vi "Record.vi"(8 "error in (no error)":errorcluster, 11 "Spectrum Recorder in":refnum<class "Spectrum Recorder.lvclass">) -> (0 "error out":errorcluster, 3 "Spectrum Recorder out":refnum<class "Spectrum Recorder.lvclass">)   [LabVIEW 2016, in "Spectrum Recorder.lvclass"]
uses:
  Spectrum Recorder.lvclass
  Spectrum Recorder.lvclass/Spectrum Recorder.ctl
  Red Pitaya/RP Core/RP Transceiver/RP Transceiver.lvclass
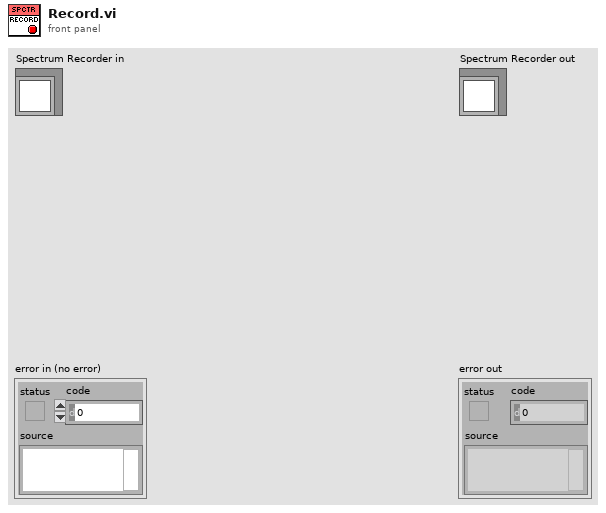
[diagram p1: front panel]
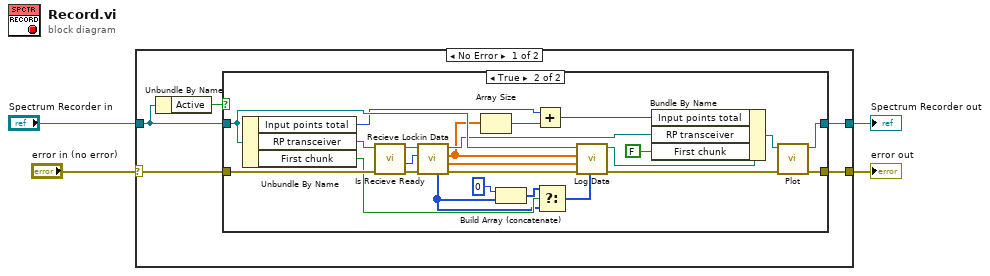
[diagram p0: block diagram]
diagram:
  n1 = case shown="No Error" "error in (no error)" {
    selector: "error in (no error)" -> [w6 w37]
    tunnel: [w5 w37] -> w3
    tunnel: [w7 w36] -> w1
    tunnel: "Spectrum Recorder in" -> [w8 w36]
    frame No Error {
      n2 = Unbundle By Name(w8) -> ("Active"=w9:bool)
      n3 = case shown="True" w9 {
        tunnel: w8 -> [w11 w28]
        tunnel: w6 -> [w10 w34]
        tunnel: [w11 w16] -> w7
        tunnel: [w10 w18] -> w5
        frame False {
        }
        frame True {
          n4 = Unbundle By Name(w28) -> ("Input points total"=w12:i64, "RP transceiver"=w35:refnum<class "RP Transceiver.lvclass">, "First chunk"=w27:bool)
          n5 = call-dynamic "Is Recieve Ready.vi"("error in (no error)"=w34, "RP Instrument in"=w35) -> ("error out"=w33:errorcluster, "Points in buffer"=w31:i32, "RP Instrument out"=w32:refnum<class "RP Transceiver.lvclass">)  [unwired: 6 in, 1 out]
          n6 = call-dynamic "Recieve Lockin Data.vi"("error in (no error)"=w33, "Points to read"=w31, "RP Lockin in"=w32) -> ("error out"=w29:errorcluster, "Volatge out"=w30:cdb[], "Frequency out"=w15:dbl[], "RP Lockin out"=w21:refnum<class "RP Transceiver.lvclass">, "Edge indexies"=w19:i32[])  [unwired: 4 in]
          n7 = Array Size(array=w15) -> (size(s)=w13:i32)
          n8 = Build Array (concatenate)(0, w19) -> (w25:i32[])
          n9 = Add(x=w12, y=w13) -> (x+y=w14:i64)
          n10 = Select(t=w25, s=w27, f=w19) -> (s? t:f=w24:i32[])
          n11 = call-dynamic "Log Data.vi"("Edge indexies"=w24, "error in (no error)"=w29, "Volatge"=w30, "Frequency"=w15, "Spectrum Recorder in"=w28) -> ("error out"=w22:errorcluster, "Spectrum Recorder out"=w23:refnum<class "Spectrum Recorder.lvclass">)  [unwired: 5 in]
          n12 = Bundle By Name(cluster=w23, "Input points total"=w14, "RP transceiver"=w21, "First chunk"=FALSE) -> (w17:refnum<class "Spectrum Recorder.lvclass">)
          n13 = call-dynamic "Plot.vi"("error in (no error)"=w22, "Spectrum Recorder in"=w17) -> ("error out"=w18:errorcluster, "Spectrum Recorder out"=w16:refnum<class "Spectrum Recorder.lvclass">)  [unwired: 8 in]
        }
      }
    }
    frame Error {
    }
  }
  "error out" <- w3
  "Spectrum Recorder out" <- w1
